vi "Introspection Core.vi"(8 "error in (no error)":errorcluster, 11 "CS++DCPwrGui in":refnum<class "CS++DCPwrGui.lvclass">) -> (0 "error out":errorcluster, 2 "CS++Messages":refnum<class "Message.lvclass">[](array[class]), 3 "CS++DCPwrGui out":refnum<class "CS++DCPwrGui.lvclass">)   [LabVIEW 2014, in "CS++DCPwrGui.lvlib" / "CS++DCPwrGui.lvclass"]
doc: "This vi delivers a list with all messages this actor reacts to. \n\nNote that all inherited classes have to overwrite it."
uses:
  CS++DCPwrGui.lvclass
  <vilib>/ActorFramework/Message/Message.lvclass
  CSPP_Core/Actors/CS++DeviceGUIActor/CS++DeviceGUIActor.lvclass
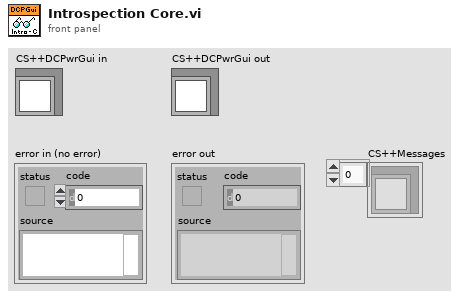
[diagram p1: front panel]
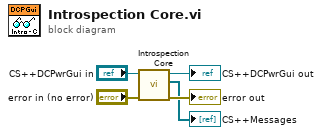
[diagram p0: block diagram]
diagram:
  n1 = call-parent "Introspection Core.vi"("error in (no error)"="error in (no error)", "CS++DeviceGUIActor in"="CS++DCPwrGui in") -> ("error out"=→"error out":errorcluster, "CS++Messages"=→"CS++Messages":refnum<class "Message.lvclass">[], "CS++DeviceGUIActor out"=→"CS++DCPwrGui out":refnum<class "CS++DCPwrGui.lvclass">)  [unwired: 7 in]
